vi "Get Item XLM String.vi"(9 "Offset In":i32, 11 "XML String":string) -> (1 "Offset Out":i32, 3 "Item XLM String":string, 7 "Finished?":bool)   [LabVIEW 2020, in "LV Project Items Parser.lvlib"]
doc: "Gets one item XLM tag and its attributes. The tabbing information will also be presented on the Item XLM String indicator. When you put this VI in a while loop and uses the Offset In and Offset out control and Indicator, you can go throug the whole project XML file. It finishes when there is no more items to retrieve in the file."
uses:
  LV Project Items Parser.lvlib
  <vilib>/regexp/Match Regular Expression.xnode
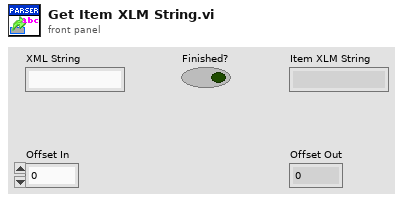
[diagram p1: front panel]
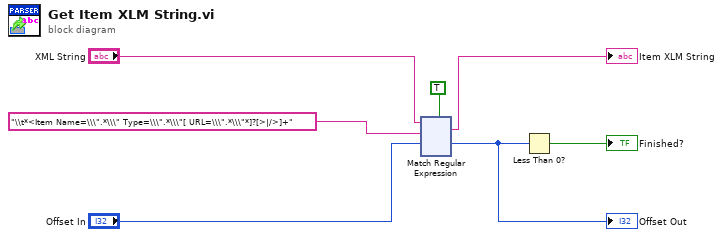
[diagram p0: block diagram]
diagram:
  n1 = xnode "Match Regular Expression"("input string"="XML String", "regular expression"="\\t*<Item Name=\\\".*\\\" Type=\\\".*\\\"[ URL=\\\".*\\\"*]?[>|/>]+" ("String"), "offset (0)"="Offset In", "multiline? (F)"=TRUE) -> ("whole match"=→"Item XLM String":string, "offset past match"=w7:i32)  [unwired: 2 in, 3 out]
  "Offset Out" <- w7
  n2 = Less Than 0?(x=w7) -> (x < 0?=→"Finished?":bool)
